vi "GetControlValue[Poly].vi"   [LabVIEW 2016, in "Drona.lvlib" / "GetControlValue.lvlib"]
doc: "Gives the value of control which is specified."
uses:
  GetControlValue/GetControlValue.lvlib
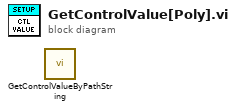
[diagram p0: block diagram]
diagram:
  n1 = call "GetControlValueByPathString.vi"() -> ()  [unwired: 13 in, 3 out]
